vi "Configure.vi"(8 "error in (no error)":errorcluster, 11 "ImageStack in":refnum<class "ImageStack.lvclass">) -> (0 "error out":errorcluster, 2 "cancelled?":bool, 3 "ImageStack out":refnum<class "ImageStack.lvclass">)   [LabVIEW 2012, in "ImageStack.lvclass"]
doc: "The configure method configures the details for the RabbitMQ connection. \n\nIn the derived class, make a call to the parent for setting these parameters."
uses:
  ImageStack.lvclass
  <vilib>/Utility/miscctls.llb/LVPointTypeDef.ctl
  ImageStack.lvclass/ImageStack.ctl
  <vilib>/Distrio/Murmex/Murmex/Murmex.lvclass
panel:
  in  "button:cancel":bool
  in  "button:configure murmex":bool
  in  "button:ok":bool
  in  "Stages component name":string
  in  "Camera component name":string
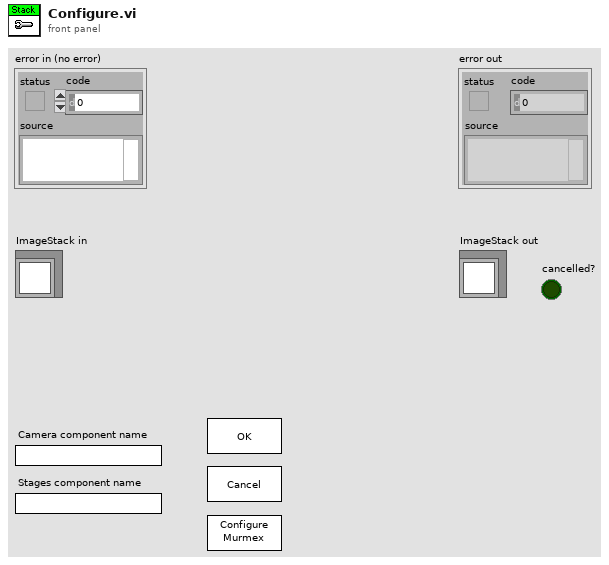
[diagram p1: front panel]
types:
  T1 = typedef "LVPointTypeDef.ctl" = cluster{"Horizontal":i16, "Vertical":i16}
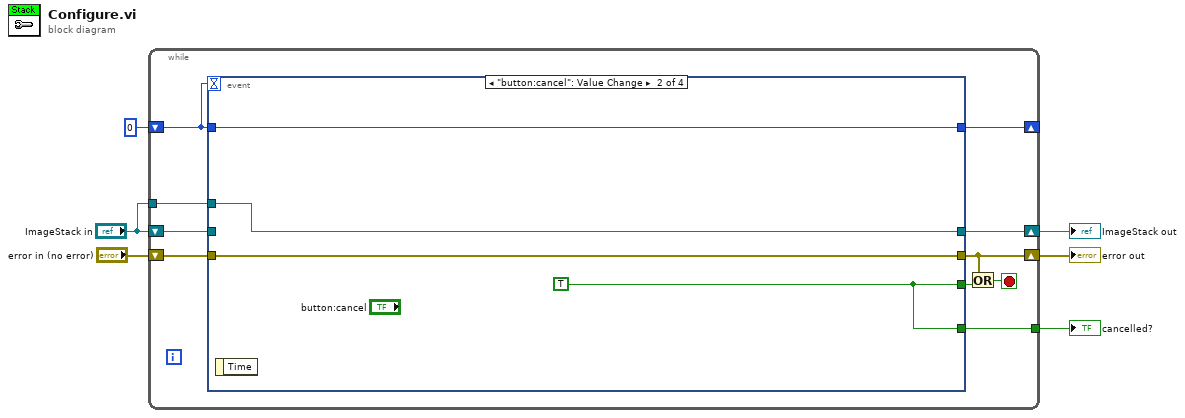
[diagram p0: block diagram]
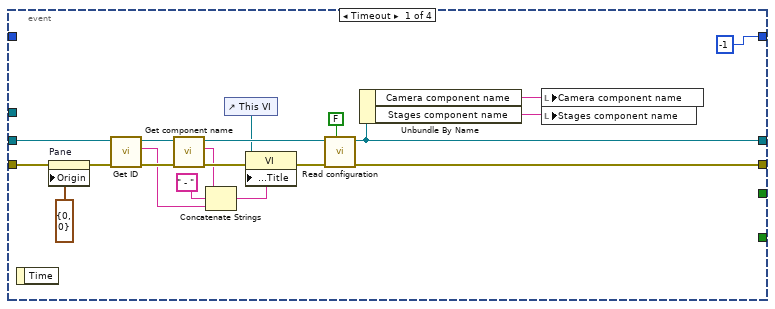
[diagram p2: hidden frame]
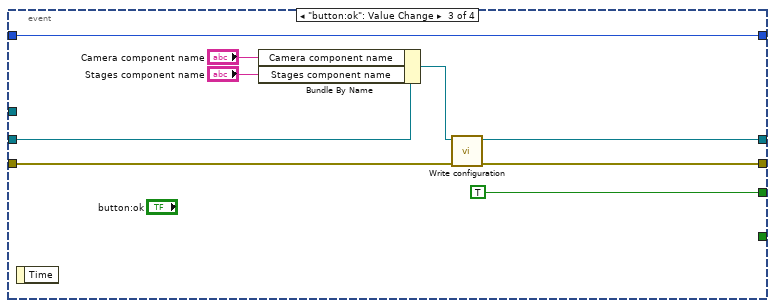
[diagram p3: hidden frame]
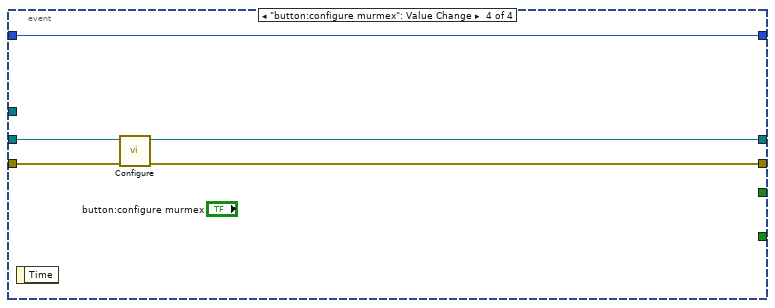
[diagram p4: hidden frame]
diagram:
  n1 = while {
    shift-right: [w11] -> w1
    shift-left: "ImageStack in" -> [w12]
    shift-right: [w13] -> w2
    shift-left: "error in (no error)" -> [w15]
    shift-right: [w16] -> _
    shift-left: 0 -> [w8]
    tunnel: "ImageStack in" -> [w9]
    tunnel: [w7] -> w3
    stop <- w14 stop-if-true
    n2 = event shown="[1] \"button:cancel\": Value Change" {
      selector: _ -> [_ _ _ _]
      dyn-events: _ -> [_ _ _ _]
      timeout: w8 -> [_ _ _ _]
      tunnel: [-1 w38 w41 w50] -> w16
      tunnel: w15 -> [w33 w40 w45 w53]
      tunnel: [w35 w40 w43 w51] -> w13
      tunnel: w12 -> [w30 _ w49 w54]
      tunnel: [w19 w39 w44 w52] -> w11
      tunnel: [_ w37 TRUE _] -> w10
      tunnel: w9 -> [_ w39 _ _]
      tunnel: w8 -> [_ w38 w41 w50]
      tunnel: [_ w37 _ _] -> w7
      event Timeout {
        n3 = event-data() -> ()  [unwired: 1 in, 1 out]
        n4 = property on="Pane" class="Pane"(error in=w33, "Origin"=T1 {"Horizontal"=0, "Vertical"=0}) -> (error out=w31:errorcluster)  [unwired: 1 in, 1 out]
        n5 = call <vilib>:"Get ID.vi"("error in (no error)"=w31, "Murmex in"=w30) -> ("error out"=w28:errorcluster, "component id"=w24:string, "Murmex out"=w29:refnum<class "ImageStack.lvclass">)  [unwired: 7 in]
        n6 = call <vilib>:"Get component name.vi"("error in (no error)"=w28, "Murmex in"=w29) -> ("error out"=w27:errorcluster, "component name"=w25:string, "Murmex out"=w26:refnum<class "ImageStack.lvclass">)  [unwired: 7 in]
        n7 = Concatenate Strings(w25, " - " ("element"), w24) -> (w20:string)
        n8 = control-ref of="This VI"() -> (w21:refnum<vi>)
        n9 = property class="VI"(reference=w21, error in=w27, "Front Panel.Title"=w20) -> (error out=w22:errorcluster)  [unwired: 1 out]
        n10 = call-dynamic "Read configuration.vi"("force loading?"=FALSE, "error in (no error)"=w22, "ImageStack in"=w26) -> ("error out"=w35:errorcluster, "ImageStack out"=w19:refnum<class "ImageStack.lvclass">)  [unwired: 7 in]
        n11 = Unbundle By Name(w19) -> ("Camera component name"=w18:string, "Stages component name"=w17:string)
        n12 = local write "Camera component name"(w18) -> ()
        n13 = local write "Stages component name"(w17) -> ()
      }
      event "button:cancel": Value Change {
        w37 = TRUE
        n14 = event-data() -> ()  [unwired: 1 in, 1 out]
      }
      event "button:ok": Value Change {
        n15 = event-data() -> ()  [unwired: 1 in, 1 out]
        n16 = Bundle By Name(cluster=w49, "Camera component name"="Camera component name", "Stages component name"="Stages component name") -> (w48:refnum<class "ImageStack.lvclass">)
        n17 = call-dynamic "Write configuration.vi"("error in (no error)"=w45, "ImageStack in"=w48) -> ("error out"=w43:errorcluster, "ImageStack out"=w44:refnum<class "ImageStack.lvclass">)  [unwired: 8 in]
      }
      event "button:configure murmex": Value Change {
        n18 = event-data() -> ()  [unwired: 1 in, 1 out]
        n19 = call-parent "Configure.vi"("error in (no error)"=w53, "Murmex in"=w54) -> ("error out"=w51:errorcluster, "Murmex out"=w52:refnum<class "ImageStack.lvclass">)  [unwired: 7 in, 1 out]
      }
    }
    n20 = Or(x=w13, y=w10) -> (x .or. y?=w14:bool)
  }
  "error out" <- w2
  "ImageStack out" <- w1
  "cancelled?" <- w3
